vi "FA_ConvertFromTDC.vi"(8 "Error In":errorcluster, 11 "TDC":T3) -> (0 "Error Out":errorcluster, 3 "Config":T1)   [LabVIEW 2014, in "FA_TDC.lvlib"]
doc: "Converts from a TDC typedef to a general config typedef"
uses:
  FA_TDC.lvlib
  FA_TDC.ctl
  FA_NativeTypes API/source/VI Source/FA_Config.ctl
  FA_LocalStore API/source/VI Source/FA_LSSpecialTypes.ctl
  FA_LocalStore API/source/VI Source/FA_LocalStore.lvlib
  FA_NativeTypes API/source/VI Source/FA_NativeTypes.lvlib
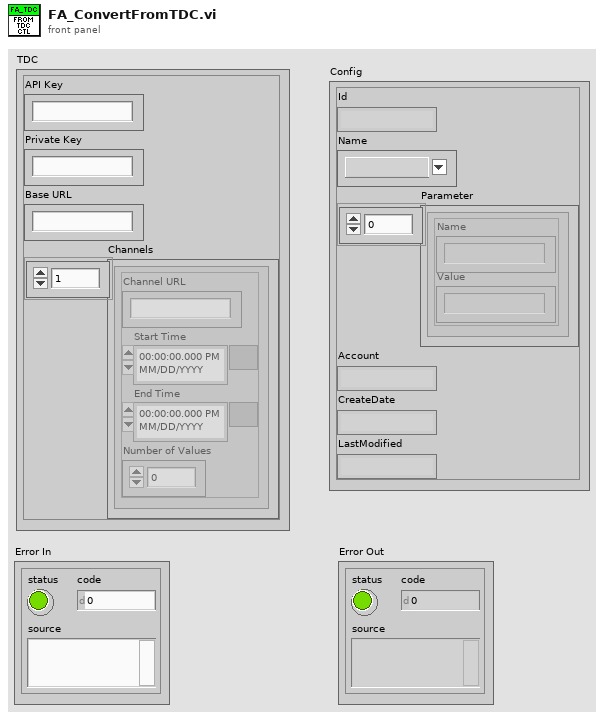
[diagram p1: front panel]
types:
  T1 = typedef "FA_NativeTypes.lvlib/FA_Config.ctl" = cluster{"Id":string, "Name":T2, "Parameter":cluster{"Name":string, "Value":string}[], "Account":string, "CreateDate":string, "LastModified":string}
  T2 = typedef "FA_LocalStore.lvlib/FA_LSSpecialTypes.ctl" = string
  T3 = typedef "FA_TDC.lvlib/FA_TDC.ctl" = cluster{"API Key":string, "Private Key":string, "Base URL":string, "Channels":cluster{"Channel URL":string, "Start Time":timestamp, "End Time":timestamp, "Number of Values":i32}[]}
  T4 = cluster{"Channel URL":string, "Start Time":timestamp, "End Time":timestamp, "Number of Values":i32}[]
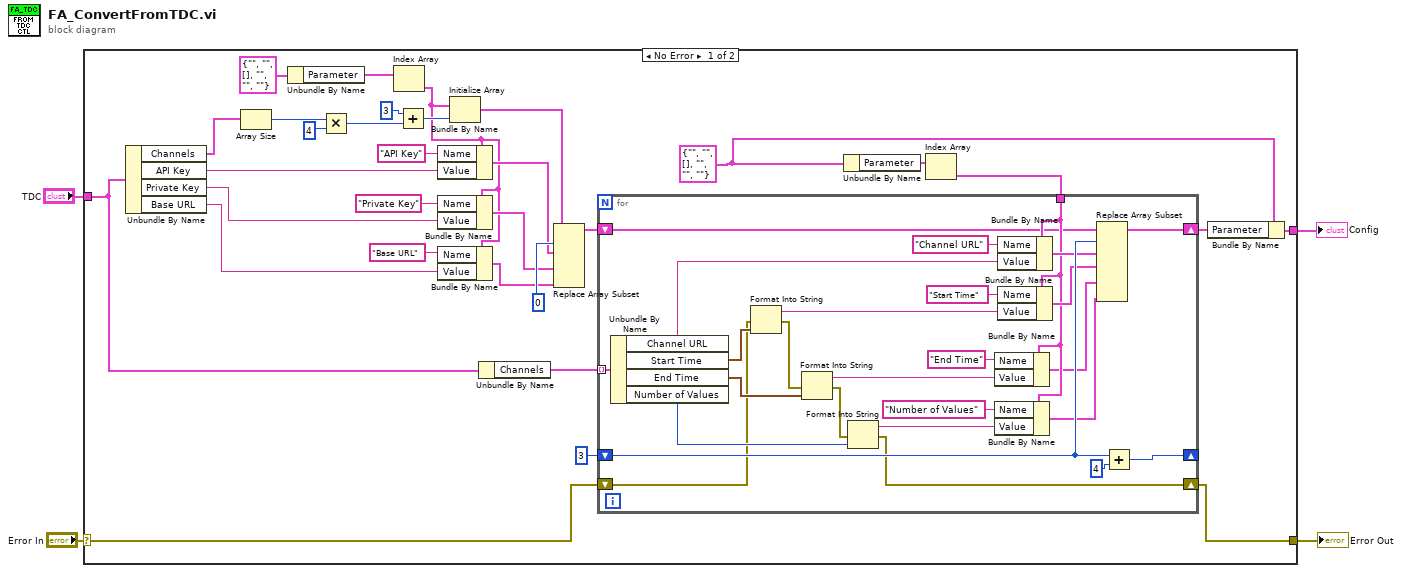
[diagram p0: block diagram]
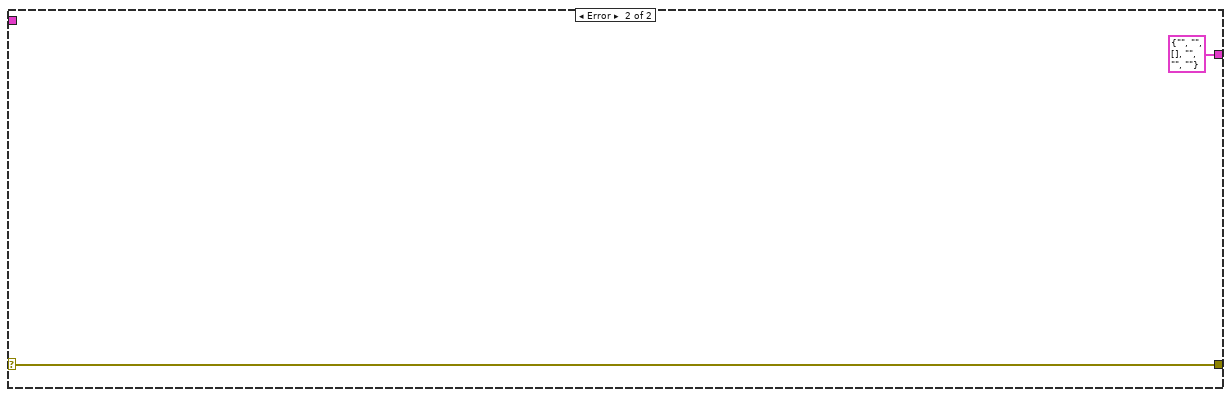
[diagram p2: hidden frame]
diagram:
  n1 = case shown="No Error" "Error In" {
    selector: "Error In" -> [w6 w62]
    tunnel: [w14 T1 {"Id"="", "Name"="", "Parameter"=[], "Account"="", "CreateDate"="", "LastModified"=""} ("Config")] -> w4
    tunnel: "TDC" -> [w11 _]
    tunnel: [w5 w62] -> w1
    frame No Error {
      w16 = T1 {"Id"="", "Name"="", "Parameter"=[], "Account"="", "CreateDate"="", "LastModified"=""} ("Config")
      n2 = Unbundle By Name(w11) -> ("Channels"=w13:T4, "API Key"=w30:string, "Private Key"=w29:string, "Base URL"=w28:string)
      n3 = Array Size(array=w13) -> (size(s)=w27:i32)
      n4 = Unbundle By Name(T1 {"Id"="", "Name"="", "Parameter"=[], "Account"="", "CreateDate"="", "LastModified"=""} ("Config")) -> ("Parameter"=w34:cluster{"Name":string, "Value":string}[])
      n5 = Multiply(x=w27, y=4) -> (x*y=w25:i32)
      n6 = Index Array(array=w34) -> (element=w7:cluster{"Name":string, "Value":string})  [unwired: 1 in]
      n7 = Add(x=3, y=w25) -> (x+y=w23:i32)
      n8 = Bundle By Name(cluster=w7, "Name"="API Key", "Value"=w30) -> (w10:cluster{"Name":string, "Value":string})
      n9 = Bundle By Name(cluster=w7, "Name"="Private Key", "Value"=w29) -> (w9:cluster{"Name":string, "Value":string})
      n10 = Bundle By Name(cluster=w7, "Name"="Base URL", "Value"=w28) -> (w8:cluster{"Name":string, "Value":string})
      n11 = Initialize Array(w7, w23) -> (w21:cluster{"Name":string, "Value":string}[])
      n12 = Unbundle By Name(w11) -> ("Channels"=w12:T4)
      n13 = Replace Array Subset(array=w21, new element #1=w10, index #1=0 ("index"), new element #2=w9, new element #3=w8) -> (w17:cluster{"Name":string, "Value":string}[])  [unwired: 2 in]
      n14 = Unbundle By Name(w16) -> ("Parameter"=w19:cluster{"Name":string, "Value":string}[])
      n15 = Index Array(array=w19) -> (element=w18:cluster{"Name":string, "Value":string})  [unwired: 1 in]
      n16 = for {
        shift-right: [w60] -> _
        shift-left: 3 ("index") -> [w59]
        tunnel: w18 -> [w52]
        shift-right: [w42] -> w15
        shift-left: w17 -> [w41]
        tunnel: w12 -> [w40] mode=indexing
        shift-right: [w36] -> w5
        shift-left: w6 -> [w39]
        n17 = Unbundle By Name(w40) -> ("Channel URL"=w58:string, "Start Time"=w48:timestamp, "End Time"=w47:timestamp, "Number of Values"=w46:i32)
        n18 = Format Into String(error in=w39, w48) -> (resulting string=w45:string, error out=w38:errorcluster)  [unwired: 2 in]
        n19 = Format Into String(error in=w38, w47) -> (resulting string=w44:string, error out=w37:errorcluster)  [unwired: 2 in]
        n20 = Format Into String(error in=w37, w46) -> (resulting string=w43:string, error out=w36:errorcluster)  [unwired: 2 in]
        n21 = Bundle By Name(cluster=w52, "Name"="End Time", "Value"=w44) -> (w51:cluster{"Name":string, "Value":string})
        n22 = Bundle By Name(cluster=w52, "Name"="Number of Values", "Value"=w43) -> (w50:cluster{"Name":string, "Value":string})
        n23 = Bundle By Name(cluster=w52, "Name"="Channel URL", "Value"=w58) -> (w54:cluster{"Name":string, "Value":string})
        n24 = Bundle By Name(cluster=w52, "Name"="Start Time", "Value"=w45) -> (w53:cluster{"Name":string, "Value":string})
        n25 = Replace Array Subset(array=w41, new element #1=w54, index #1=w59, new element #2=w53, new element #3=w51, new element #4=w50) -> (w42:cluster{"Name":string, "Value":string}[])  [unwired: 3 in]
        n26 = Add(x=w59, y=4) -> (x+y=w60:i32)
      }
      n27 = Bundle By Name(cluster=w16, "Parameter"=w15) -> (w14:T1)
    }
    frame Error {
    }
  }
  "Error Out" <- w1
  "Config" <- w4
